vi "Get all Object Items (fixup).vi"(8 "error in (no error)":errorcluster, 10 "Offset":i32, 11 "JSON":string) -> (0 "error out":errorcluster, 1 "<JSON>":string[](array[string]) caption="<JSON>Items", 2 "Offset past":i32 caption="Offset past Object", 3 "Item Names":string[](array[string]))   [LabVIEW 2019]
doc: "Return all Items in the Object as an array of JSON Values."
uses:
  Parsing/Parsing State.ctl
  JSONtext.lvlib
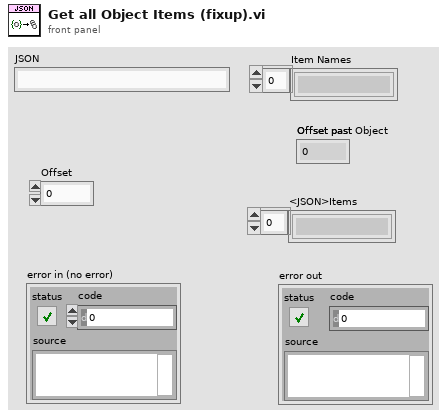
[diagram p1: front panel]
types:
  T1 = typedef "JSONtext.lvlib/Parsing State.ctl" = enum16{"Parser Error", "Object", "Array", "String", "Number/Other", "Leading Whitespace", "Object end", "Array end", "Value end"}
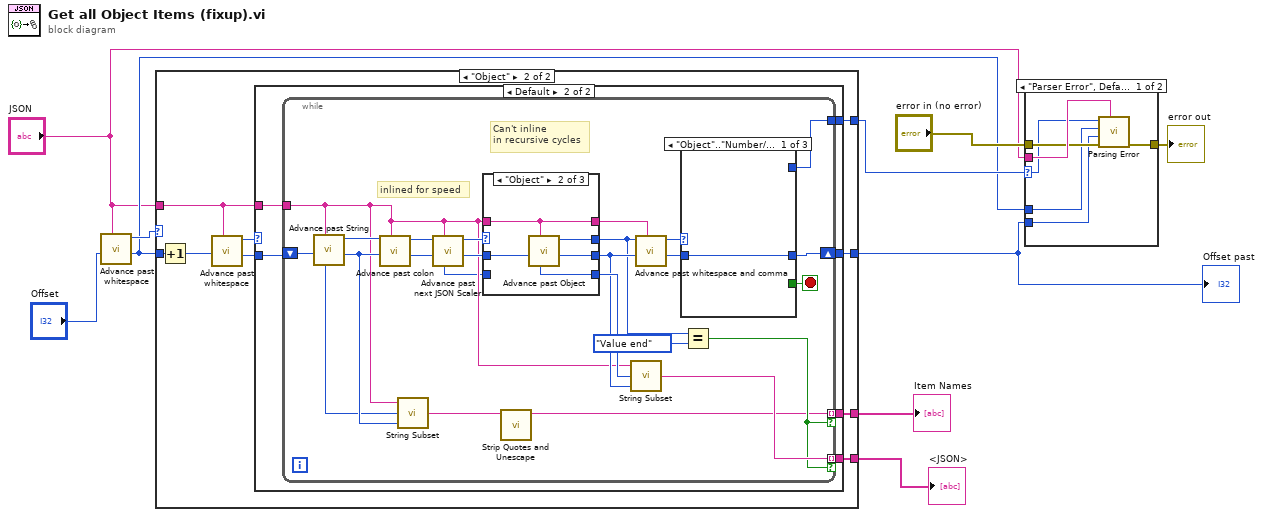
[diagram p0: block diagram]
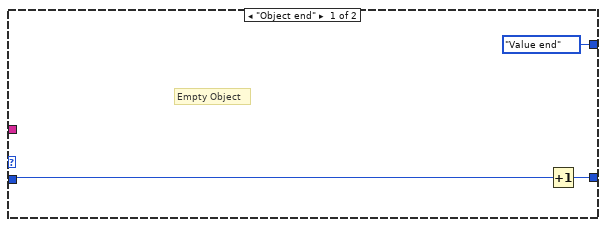
[diagram p3: hidden frame]
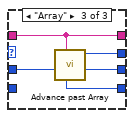
[diagram p5: hidden frame]
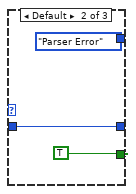
[diagram p6: hidden frame]
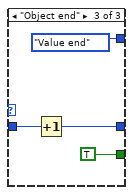
[diagram p7: hidden frame]
diagram:
  n1 = call "Advance past whitespace.vi"("JSON"="JSON", "Offset"="Offset") -> ("Offset of first non-whitespace"=w2:i32, "Parser State"=w7:T1)  [unwired: 7 in, 1 out]
  n2 = case shown="\"Object\"" w7 {
    selector: w7 -> [w12 _]
    tunnel: [w12 w21] -> w3
    tunnel: [_ w20] -> w10
    tunnel: [_ w19] -> w9
    tunnel: w2 -> [w11 w18]
    tunnel: "JSON" -> [_ w14]
    tunnel: [w11 w17] -> w4
    frame "Parser Error", Default {
    }
    frame "Object" {
      n3 = Increment(x=w18) -> (x+1=w16:i32)
      n4 = call "Advance past whitespace.vi"("JSON"=w14, "Offset"=w16) -> ("Offset of first non-whitespace"=w15:i32, "Parser State"=w13:T1)  [unwired: 7 in, 1 out]
      n5 = case shown="Default" w13 {
        tunnel: [Parsing_State."Value end" w30] -> w21
        tunnel: [_ w29] -> w20
        tunnel: [_ w28] -> w19
        tunnel: [w23 w27] -> w17
        tunnel: w15 -> [w22 w26]
        tunnel: w14 -> [_ w25]
        frame "Object end" {
          # "Empty Object"
          n6 = Increment(x=w22) -> (x+1=w23:i32)
        }
        frame Default {
          n7 = while {
            shift-right: [w51] -> w27
            shift-left: w26 -> [w31]
            tunnel: w25 -> [w40]
            tunnel: [w49] -> w30
            tunnel: [w34] -> w29 mode=indexing if=w36
            tunnel: [w39] -> w28 mode=indexing if=w36
            stop <- w50 stop-if-true
            # "Can't inline\nin recursive cycles"
            # "inlined for speed"
            n8 = call "Advance past String.vi"("JSON"=w40, "Offset"=w31) -> ("Offset past match"=w43:i32, "State"=w54:T1, "Value start out"=w33:i32)  [unwired: 7 in]
            n9 = call "Advance past colon.vi"("JSON"=w40, "Offset"=w43, "State"=w54) -> ("index"=w45:i32, "State"=w46:T1)  [unwired: 7 in]
            n10 = call "String Subset.vi"("Offset past End"=w43, "Start offset"=w33, "JSON"=w40) -> ("substring"=w35:string)  [unwired: 2 in]
            n11 = call "Advance past next JSON Scaler.vi"("JSON"=w40, "Offset"=w45, "Parser State in"=w46) -> ("Offset Past"=w44:i32, "Parser State"=w47:T1, "Value start"=w32:i32)  [unwired: 6 in]
            n12 = case shown="\"Object\"" w47 {
              selector: w47 -> [w57 _ _]
              tunnel: w44 -> [w56 w63 w68]
              tunnel: [w57 w62 w67] -> w38
              tunnel: [w56 w61 w66] -> w41
              tunnel: w40 -> [w58 w60 w65]
              tunnel: [w58 w60 w65] -> w48
              tunnel: [w55 w59 w64] -> w42
              tunnel: w32 -> [w55 _ _]
              frame Default {
              }
              frame "Object" {
                n13 = call "Advance past Object.vi"("JSON"=w60, "Offset"=w63) -> ("Offset past Object"=w61:i32, "State"=w62:T1, "Object Start"=w59:i32)  [unwired: 7 in]
              }
              frame "Array" {
                n14 = call "Advance past Array.vi"("JSON"=w65, "Offset"=w68) -> ("Offset past Array"=w66:i32, "State"=w67:T1, "Array Start"=w64:i32)  [unwired: 6 in, 1 out]
              }
            }
            n15 = call "Strip Quotes and Unescape.vi"("String"=w35) -> ("result string"=w34:string)  [unwired: 9 in, 1 out]
            n16 = call "String Subset.vi"("Offset past End"=w41, "Start offset"=w42, "JSON"=w40) -> ("substring"=w39:string)  [unwired: 2 in]
            n17 = call "Advance past whitespace and comma.vi"("JSON"=w48, "Offset"=w41, "State in"=w38) -> ("Offset past match"=w53:i32, "State"=w52:T1)  [unwired: 6 in, 1 out]
            n18 = case shown="\"Object\"..\"Number/Other\"" w52 {
              tunnel: [_ TRUE TRUE] -> w50
              tunnel: [_ Parsing_State."Parser Error" Parsing_State."Value end"] -> w49
              tunnel: w53 -> [w69 w70 w74]
              tunnel: [w69 w70 w73] -> w51
              frame "Object".."Number/Other" {
              }
              frame Default {
              }
              frame "Object end" {
                n19 = Increment(x=w74) -> (x+1=w73:i32)
              }
            }
            n20 = Equal?(x=w38, y=Parsing_State."Value end") -> (x = y?=w36:bool)
          }
        }
      }
    }
  }
  "Item Names" <- w10
  "<JSON>" <- w9
  "Offset past" <- w4
  n21 = case shown="\"Parser Error\", Default" w3 {
    selector: w3 -> [w77 _]
    tunnel: "JSON" -> [w82 _]
    tunnel: "error in (no error)" -> [w81 w83]
    tunnel: [w80 w83] -> w6
    tunnel: w2 -> [w79 _]
    tunnel: w4 -> [w78 _]
    frame "Parser Error", Default {
      n22 = call "Parsing Error.vi"("JSON"=w82, "error in (no error)"=w81, "Offset past match"=w78, "Value start"=w79, "State"=w77) -> ("error out"=w80:errorcluster)  [unwired: 6 in]
    }
    frame "Value end" {
    }
  }
  "error out" <- w6
